vi "Filter Control Drag Over Event.vi"(8 "error in (no error)":errorcluster, 10 "ControlDragOverMsg":refnum<class "ControlDragOverMsg.lvclass">, 11 "Test Executive Builder Event Filter in":refnum<class "Test Executive Builder Event Filter.lvclass">) -> (0 "error out":errorcluster, 1 "Discard?":bool, 3 "Test Executive Builder Event Filter out":refnum<class "Test Executive Builder Event Filter.lvclass">)   [LabVIEW 2017, in "Test Executive Builder Event Filter.lvclass"]
uses:
  Test Executive Builder Event Filter.lvclass
  <vilib>/gpm_packages/@cs/mva-viewable/Source/ActorEvents/IEventAggregator Messages/ControlDragOverMsg/ControlDragOverMsg.lvclass
  Test Executive Builder View Messages/Handle Drag Over Msg/Handle Drag Over Msg.lvclass
  <vilib>/gpm_packages/@cs/actor-framework-messages/Source/RoundTripMessage/RoundTripMessage.lvclass
  C:/Users/jonmc/Documents/Git/Test Executive Builder/gpm_packages/@cs/actor-framework-messages/Source/RoundTripMessage/RoundTripMessage.lvclass
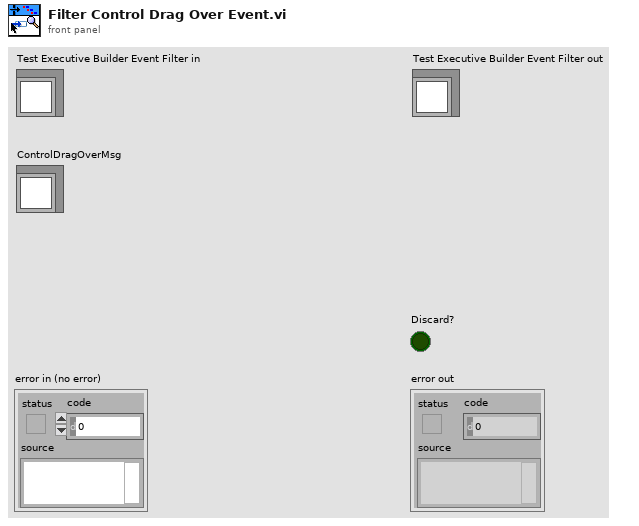
[diagram p1: front panel]
types:
  T1 = typedef "LVPoint32TypeDef.ctl" = cluster{"Horizontal":i32, "Vertical":i32}
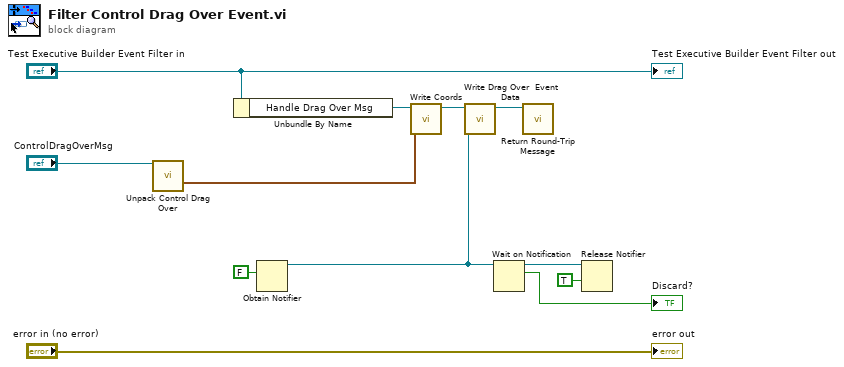
[diagram p0: block diagram]
diagram:
  n1 = call <vilib>:"Unpack Control Drag Over.vi"("ControlDragOverMsg In"="ControlDragOverMsg") -> ("Coords"=w3:T1)  [unwired: 7 in, 7 out]
  n2 = Unbundle By Name("Test Executive Builder Event Filter in") -> ("Handle Drag Over Msg"=w5:refnum<class "Handle Drag Over Msg.lvclass">)
  n3 = Obtain Notifier(notification data type=FALSE) -> (notifier out=w2:refnum<notifier>)  [unwired: 3 in, 2 out]
  n4 = call "Write Coords.vi"("Coordinates"=w3, "Handle Drag Over Msg in"=w5) -> ("Handle Drag Over Msg out"=w4:refnum<class "Handle Drag Over Msg.lvclass">)  [unwired: 9 in]
  n5 = call "Write Drag Over  Event Data.vi"("Drag Over  Event Data"=w2, "Handle Drag Over Msg in"=w4) -> ("Handle Drag Over Msg out"=w1:refnum<class "Handle Drag Over Msg.lvclass">)  [unwired: 9 in]
  n6 = Wait on Notification(notifier=w2) -> (notifier out=w9:refnum<notifier>, notification=→"Discard?":bool)  [unwired: 3 in, 2 out]
  n7 = call <vilib>:"Return Round-Trip Message.vi"("RoundTripMessage In"=w1) -> ()  [unwired: 10 in, 1 out]
  n8 = Release Notifier(notifier=w9, force destroy? (F)=TRUE) -> ()  [unwired: 1 in, 3 out]
  "error out" <- "error in (no error)"
  "Test Executive Builder Event Filter out" <- "Test Executive Builder Event Filter in"
